vi "Tick Period to Speed.vi"(9 "Tire Diameter (m)":dbl, 10 "Boolean":bool, 11 "Tick Period":dbl) -> (3 "Wheel Speed (m/s)":dbl)   [LabVIEW 2014]
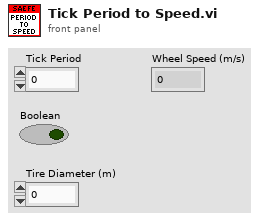
[diagram p1: front panel]
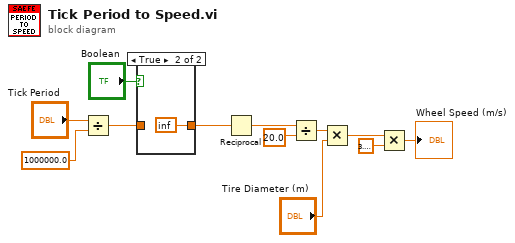
[diagram p0: block diagram]
diagram:
  n1 = Divide(x="Tick Period", y=1000000.0) -> (x/y=w3:dbl)
  n2 = case shown="True" "Boolean" {
    tunnel: w3 -> [w13 _]
    tunnel: [w13 inf] -> w12
    frame False {
    }
    frame True {
    }
  }
  n3 = Reciprocal(x=w12) -> (1/x=w4:dbl)
  n4 = Divide(x=w4, y=20.0) -> (x/y=w6:dbl)
  n5 = Multiply(x=w6, y="Tire Diameter (m)") -> (x*y=w8:dbl)
  n6 = Multiply(x=w8, y=3.141592653589793) -> (x*y=→"Wheel Speed (m/s)":dbl)
